vi "Draw GUI running average centroid overlay.vi"(8 "error in":errorcluster, 10 "GUI_centroid overlay":T1={"CentroidX array"=[], "CentroidY array"=[], "CentroidX"=0.0, "CentroidY"=0.0, "# images to average"=1250067, "Crosshair"={"Draw"=TRUE, "Target"={"x"=20.0, "y"=20.0}, "Size"={"x"=20.0, "y"=20.0}, "Angle"=1250067.0, "Color"=1250067, "Thickness"=20, "CrosshairLabel"=""}} {"Crosshair"."Thickness" max=0; "Crosshair"."Target"."y" min=0.0 max=0.0; "Crosshair"."Target"."x" min=0.0 max=0.0; "Crosshair"."Angle" format="%#_13g"; "Crosshair"."Size"."y" min=0.0 max=0.0; "Crosshair"."Size"."x" min=0.0 max=0.0}, 11 "Image in":T3) -> (0 "error out":errorcluster, 3 "image out":T3)   [LabVIEW 2013]
doc: "Draw Crosshair in image as per targetx and y and size\ninput:\n1. Draw crosshair cluster (Image in, Draw(boolean), size, target x, target y)\n2. Error in\noutput\n1.Error out"
uses:
  <vilib>/vision/Image Controls.llb/IMAQ Image.ctl
  Controls/GUI_running average centroid overlay.ctl
  Controls/Crosshair type def.ctl
  <vilib>/ptbypt/NI_PtbyPt.lvlib
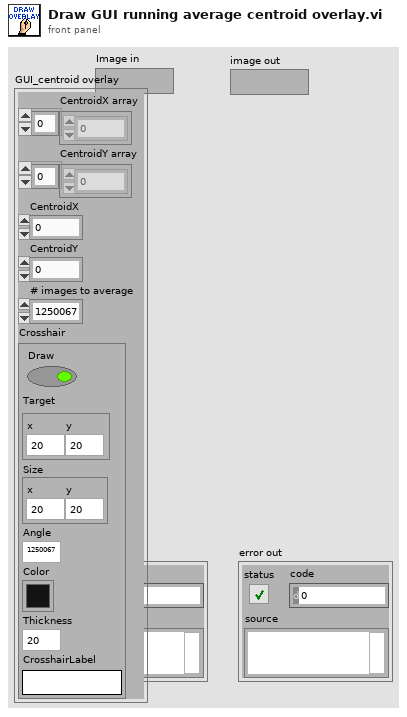
[diagram p1: front panel]
types:
  T1 = typedef "GUI_running average centroid overlay.ctl" = cluster{"CentroidX array":dbl[], "CentroidY array":dbl[], "CentroidX":dbl, "CentroidY":dbl, "# images to average":i32, "Crosshair":T2}
  T2 = typedef "Crosshair type def.ctl" = cluster{"Draw":bool, "Target":cluster{"x":dbl, "y":dbl}, "Size":cluster{"x":dbl, "y":dbl}, "Angle":dbl, "Color":u32, "Thickness":u8, "CrosshairLabel":string}
  T3 = typedef "IMAQ Image.ctl" = refnum<image>
  T4 = cluster{"Left":i32, "Top":i32, "Right":i32, "Bottom":i32}
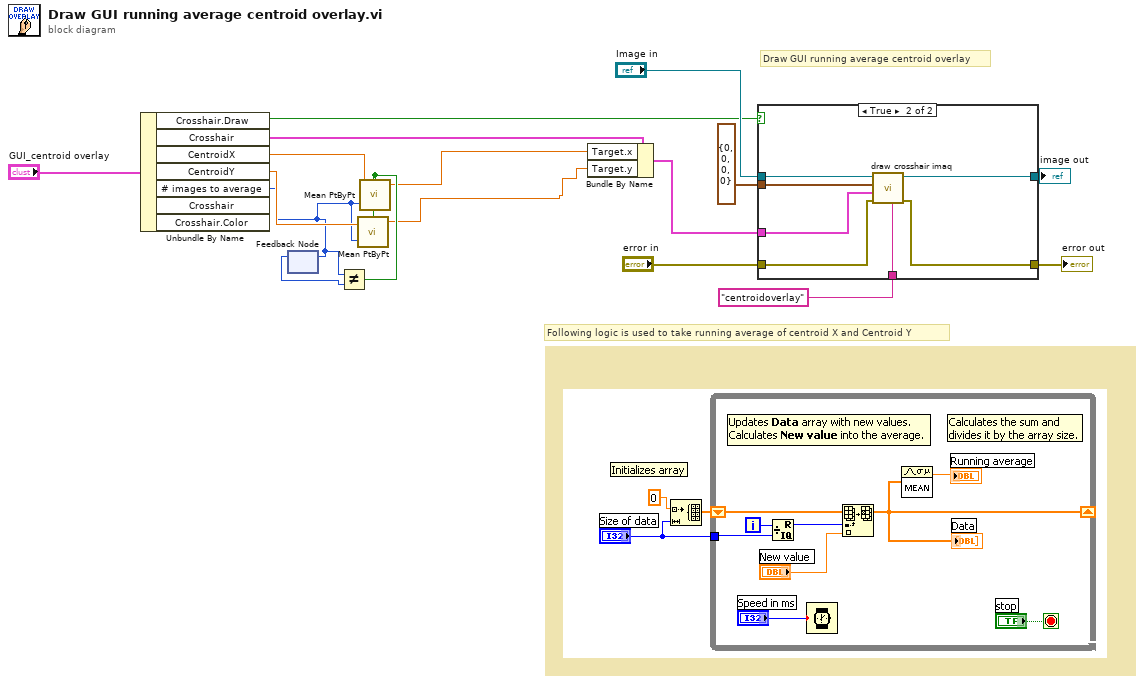
[diagram p0: block diagram]
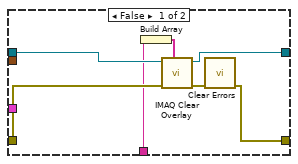
[diagram p2: hidden frame]
diagram:
  # "Following logic is used to take running average of centroid X and Centroid Y"
  # "Draw GUI running average centroid overlay"
  n1 = Unbundle By Name("GUI_centroid overlay") -> ("Crosshair.Draw"=w11:bool, "Crosshair"=w4:T2, "CentroidX"=w9:dbl, "CentroidY"=w8:dbl, "# images to average"=w7:i32)  [unwired: 2 out]
  n2 = feedback-in #1(w7) -> ()
  n3 = feedback #1() -> (w6:i32)  [unwired: 1 in]
  n4 = Not Equal?(x=w7, y=w6) -> (x != y?=w5:bool)
  n5 = call <vilib>:"Mean PtByPt.vi"("x"=w8, "sample length"=w7, "initialize"=w5) -> ("mean"=w2:dbl)  [unwired: 1 in, 1 out]
  n6 = call <vilib>:"Mean PtByPt.vi"("x"=w9, "sample length"=w7, "initialize"=w5) -> ("mean"=w3:dbl)  [unwired: 1 in, 1 out]
  n7 = Bundle By Name(cluster=w4, "Target.x"=w3, "Target.y"=w2) -> (w1:T2)
  n8 = case shown="True" w11 {
    tunnel: "Image in" -> [w24 w31]
    tunnel: [w23 w29] -> w13
    tunnel: T4 {"Left"=0, "Top"=0, "Right"=0, "Bottom"=0} ("Bounding Rectangle") -> [_ w30]
    tunnel: "error in" -> [w22 w28]
    tunnel: [w21 w27] -> w16
    tunnel: "centroidoverlay" ("overlay name") -> [w18 w26]
    tunnel: w1 -> [_ w25]
    frame False {
      n9 = Build Array(w18) -> (w19:string[])
      n10 = call "IMAQ Clear Overlay"("Groups"=w19, "error in (no error)"=w22, "Image"=w24) -> ("error out"=w20:errorcluster, "Image Out"=w23:T3)  [unwired: 7 in]
      n11 = call <vilib>:"Clear Errors.vi"("error in (no error)"=w20) -> ("error out"=w21:errorcluster)  [unwired: 6 in]
    }
    frame True {
      n12 = call "draw crosshair imaq.vi"("overlay name"=w26, "error in (no error)"=w28, "Crosshair"=w25, "Bounding Rectangle"=w30, "image in"=w31) -> ("error out"=w27:errorcluster, "image out"=w29:T3)  [unwired: 5 in]
    }
  }
  "error out" <- w16
  "image out" <- w13
